vi "Calculate Timing Characteristics.vi"(10 "Engine Clock Rate (MHz)":i32=120000000 format="%.0p", 11 "SPI Signals":T2) -> (3 "Timing Characteristics":T1)   [LabVIEW 2014]
uses:
  Controls/Digital Data.ctl
  Controls/Timing Characteristics.ctl
panel:
  out "CS Rising Tick":i32
  out "tCSH (Ticks)":i32
  out "tCSH (ns)":dbl format="%#.2f"
  out "SCLK Frequency":dbl format="%.2p"
  out "tCP (ns)":dbl format="%#.2f"
  out "SCLK Rising Tick":i32
  out "First SCLK Tick":i32
  out "tCSS (Ticks)":i32
  out "tCSS (ns)":dbl format="%#.2f"
  out "SCLK Falling Tick":i32
  out "SCLK Falling Tick (Prev)":i32
  out "Actual Rate (S/s)":dbl format="%#.2p"
  out "CS Falling Period":i32
  out "CS Falling Tick":i32
  out "tCSW (Ticks)":i32
  out "tCSW (ns)":dbl format="%#.2f"
  out "Simulation Tick":i32
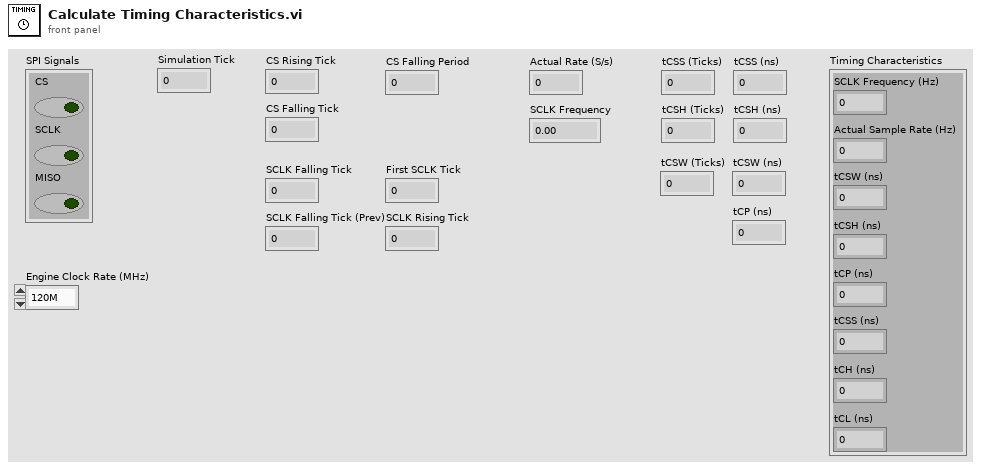
[diagram p1: front panel]
types:
  T1 = typedef "Timing Characteristics.ctl" = cluster{"SCLK Frequency (Hz)":dbl, "Actual Sample Rate (Hz)":dbl, "tCSW (ns)":dbl, "tCSH (ns)":dbl, "tCSS (ns)":dbl, "tCP (ns)":dbl, "tCH (ns)":dbl, "tCL (ns)":dbl}
  T2 = typedef "Digital Data.ctl" = cluster{"CS":bool, "SCLK":bool, "MISO":bool}
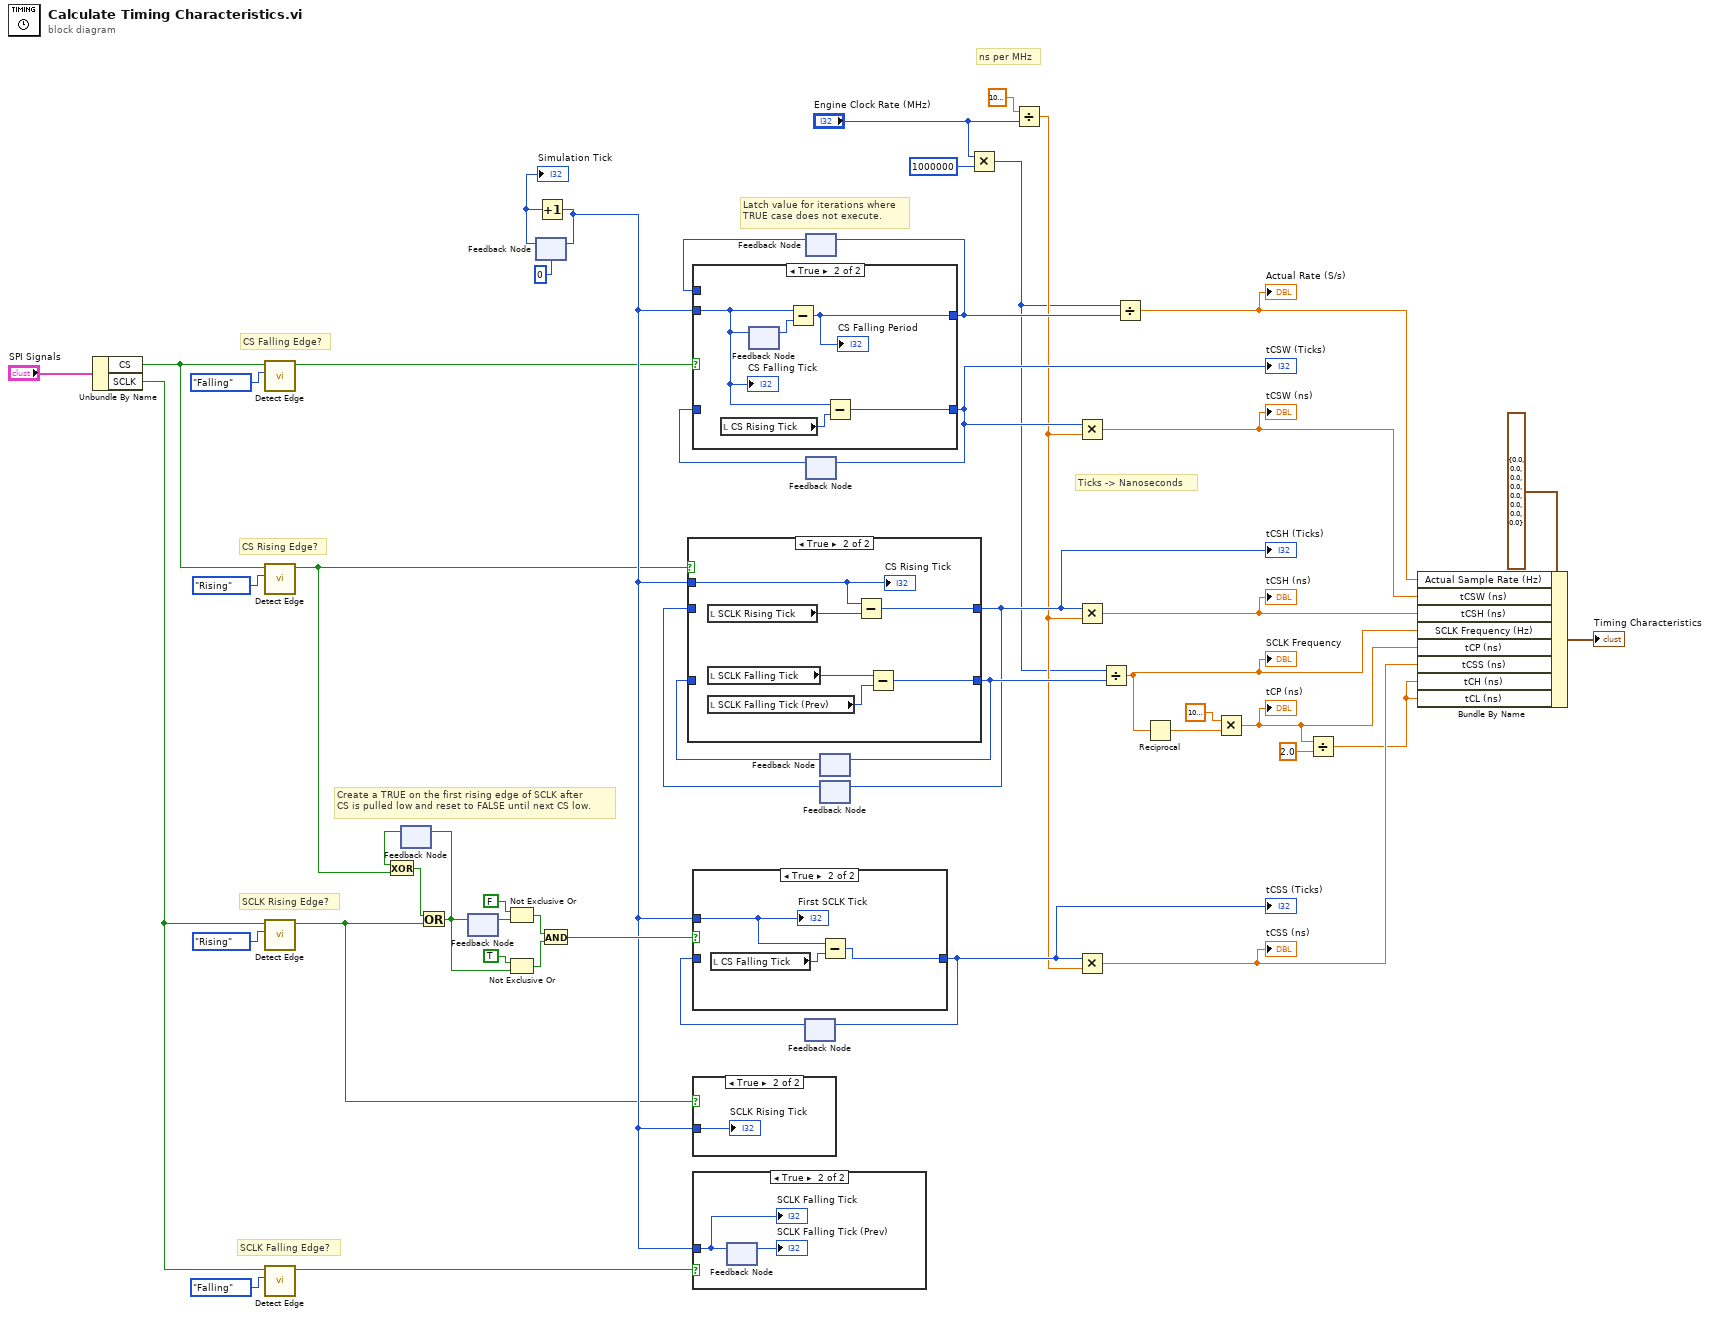
[diagram p0: block diagram]
diagram:
  # "ns per MHz"
  # "Ticks -> Nanoseconds"
  # "Latch value for iterations where\nTRUE case does not execute."
  # "SCLK Falling Edge?"
  # "SCLK Rising Edge?"
  # "CS Rising Edge?"
  # "CS Falling Edge?"
  # "Create a TRUE on the first rising edge of SCLK after\nCS is pulled low and reset to FALSE until next CS low."
  n1 = Unbundle By Name("SPI Signals") -> ("CS"=w21:bool, "SCLK"=w24:bool)
  n2 = call "Detect Edge.vi"("Edge Type?"=enum16{"Rising", "Falling"}."Falling", "Signal In"=w21) -> ("Edge Detected?"=w29:bool)  [unwired: 9 in]
  n3 = call "Detect Edge.vi"("Edge Type?"=enum16{"Rising", "Falling"}."Rising", "Signal In"=w21) -> ("Edge Detected?"=w27:bool)  [unwired: 9 in]
  n4 = call "Detect Edge.vi"("Edge Type?"=enum16{"Rising", "Falling"}."Rising", "Signal In"=w24) -> ("Edge Detected?"=w22:bool)  [unwired: 9 in]
  n5 = call "Detect Edge.vi"("Edge Type?"=enum16{"Rising", "Falling"}."Falling", "Signal In"=w24) -> ("Edge Detected?"=w23:bool)  [unwired: 9 in]
  n6 = feedback #1() -> (w47:bool)  [unwired: 1 in]
  n7 = Exclusive Or(1:w27, 2:w47) -> (0:w46:bool)
  n8 = Or(x=w46, y=w22) -> (x .or. y?=w42:bool)
  n9 = feedback-in #1(w42) -> ()
  n10 = feedback #2() -> (w43:bool)  [unwired: 1 in]
  n11 = feedback-in #2(w42) -> ()
  n12 = Not Exclusive Or(1:w43, 2:FALSE ("x")) -> (0:w41:bool)
  n13 = Not Exclusive Or(1:w42, 2:TRUE ("x")) -> (0:w40:bool)
  n14 = feedback #3(0 ("Simulation Ticks")) -> (w48:i32)
  "Simulation Tick" <- w48
  n15 = Increment(x=w48) -> (x+1=w38:i32)
  n16 = feedback-in #3(w38) -> ()
  n17 = And(x=w41, y=w40) -> (x .and. y?=w39:bool)
  n18 = case shown="True" w22 {
    tunnel: w38 -> [_ w51]
    frame False {
    }
    frame True {
      "SCLK Rising Tick" <- w51
    }
  }
  n19 = case shown="True" w23 {
    tunnel: w38 -> [_ w52]
    frame False {
    }
    frame True {
      n20 = feedback #4() -> (→"SCLK Falling Tick (Prev)":i32)  [unwired: 1 in]
      n21 = feedback-in #4(w52) -> ()
      "SCLK Falling Tick" <- w52
    }
  }
  n22 = feedback #5() -> (w31:i32)  [unwired: 1 in]
  n23 = case shown="True" w39 {
    tunnel: w38 -> [_ w56]
    tunnel: [w54 w55] -> w19
    tunnel: w31 -> [w54 _]
    frame False {
    }
    frame True {
      n24 = local read "CS Falling Tick"() -> (w57:i32)
      n25 = Subtract(x=w56, y=w57) -> (x-y=w55:i32)
      "First SCLK Tick" <- w56
    }
  }
  "tCSS (Ticks)" <- w19
  n26 = feedback-in #5(w19) -> ()
  n27 = feedback #6() -> (w15:i32)  [unwired: 1 in]
  n28 = feedback #7() -> (w37:i32)  [unwired: 1 in]
  n29 = case shown="True" w29 {
    tunnel: w38 -> [_ w61]
    tunnel: [w59 w62] -> w18
    tunnel: w37 -> [w59 _]
    tunnel: [w58 w60] -> w14
    tunnel: w15 -> [w58 _]
    frame False {
    }
    frame True {
      n30 = local read "CS Rising Tick"() -> (w64:i32)
      n31 = feedback-in #8(w61) -> ()
      n32 = feedback #8() -> (w63:i32)  [unwired: 1 in]
      n33 = Subtract(x=w61, y=w63) -> (x-y=w60:i32)
      "CS Falling Period" <- w60
      n34 = Subtract(x=w61, y=w64) -> (x-y=w62:i32)
      "CS Falling Tick" <- w61
    }
  }
  "tCSW (Ticks)" <- w18
  n35 = feedback-in #6(w14) -> ()
  n36 = feedback-in #7(w18) -> ()
  n37 = feedback #9() -> (w33:i32)  [unwired: 1 in]
  n38 = feedback #10() -> (w32:i32)  [unwired: 1 in]
  n39 = case shown="True" w27 {
    tunnel: w38 -> [_ w69]
    tunnel: [w65 w68] -> w20
    tunnel: [w66 w67] -> w34
    tunnel: w33 -> [w66 _]
    tunnel: w32 -> [w65 _]
    frame False {
    }
    frame True {
      n40 = local read "SCLK Rising Tick"() -> (w72:i32)
      n41 = local read "SCLK Falling Tick"() -> (w71:i32)
      n42 = local read "SCLK Falling Tick (Prev)"() -> (w70:i32)
      n43 = Subtract(x=w69, y=w72) -> (x-y=w68:i32)
      n44 = Subtract(x=w71, y=w70) -> (x-y=w67:i32)
      "CS Rising Tick" <- w69
    }
  }
  "tCSH (Ticks)" <- w20
  n45 = feedback-in #9(w34) -> ()
  n46 = feedback-in #10(w20) -> ()
  n47 = Multiply(x="Engine Clock Rate (MHz)", y=1000000) -> (x*y=w2:i32)
  n48 = Divide(x=1000.0, y="Engine Clock Rate (MHz)") -> (x/y=w4:dbl)
  n49 = Multiply(x=w18, y=w4) -> (x*y=w13:dbl)
  "tCSW (ns)" <- w13
  n50 = Multiply(x=w20, y=w4) -> (x*y=w11:dbl)
  "tCSH (ns)" <- w11
  n51 = Multiply(x=w19, y=w4) -> (x*y=w10:dbl)
  "tCSS (ns)" <- w10
  n52 = Divide(x=w2, y=w34) -> (x/y=w9:dbl)
  "SCLK Frequency" <- w9
  n53 = Divide(x=w2, y=w14) -> (x/y=w12:dbl)
  "Actual Rate (S/s)" <- w12
  n54 = Reciprocal(x=w9) -> (1/x=w36:dbl)
  n55 = Multiply(x=1000000000.0, y=w36) -> (x*y=w8:dbl)
  "tCP (ns)" <- w8
  n56 = Divide(x=w8, y=2.0) -> (x/y=w6:dbl)
  n57 = Bundle By Name(cluster=T1 {"SCLK Frequency (Hz)"=0.0, "Actual Sample Rate (Hz)"=0.0, "tCSW (ns)"=0.0, "tCSH (ns)"=0.0, "tCSS (ns)"=0.0, "tCP (ns)"=0.0, "tCH (ns)"=0.0, "tCL (ns)"=0.0} ("input cluster"), "Actual Sample Rate (Hz)"=w12, "tCSW (ns)"=w13, "tCSH (ns)"=w11, "SCLK Frequency (Hz)"=w9, "tCP (ns)"=w8, "tCSS (ns)"=w10, "tCH (ns)"=w6, "tCL (ns)"=w6) -> (→"Timing Characteristics":T1)
